vi "Init.vi"(2 "Value":refnum<class>, 3 "Which Index":i32) -> (1 "Action out":refnum<class "Act_Set One.lvclass">)   [LabVIEW 2014, in "Act_Set One.lvclass"]
uses:
  Act_Set One.lvclass
  Act_Set One.lvclass/Act_Set One.ctl
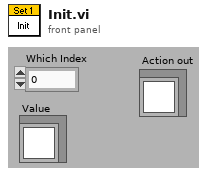
[diagram p1: front panel]
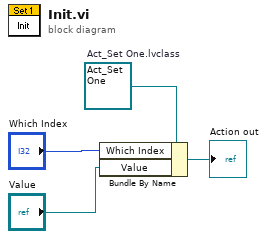
[diagram p0: block diagram]
diagram:
  w4 = refnum<class "Act_Set One.lvclass"> refnum  # Act_Set One.lvclass
  n1 = Bundle By Name(cluster=w4, "Which Index"="Which Index", "Value"="Value") -> (→"Action out":refnum<class "Act_Set One.lvclass">)
